vi "Variant to ITX Wave.vi"(8 "error in (no error)":errorcluster, 10 "Data":variant, 11 "Wavename":string) -> (0 "error out":errorcluster, 3 "ITX Wave":string)   [LabVIEW 2019, in "LV-Data.ITX.lvclass"]
uses:
  LV-Data.ITX.lvclass
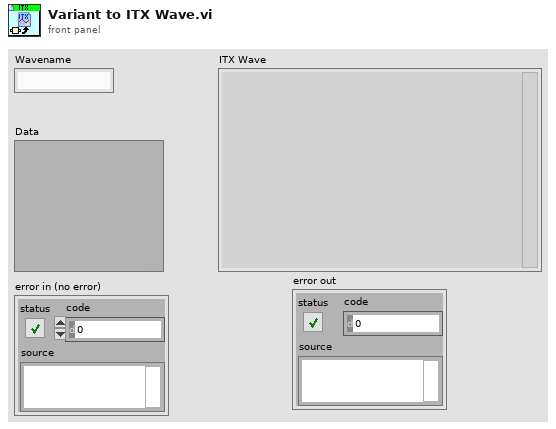
[diagram p1: front panel]
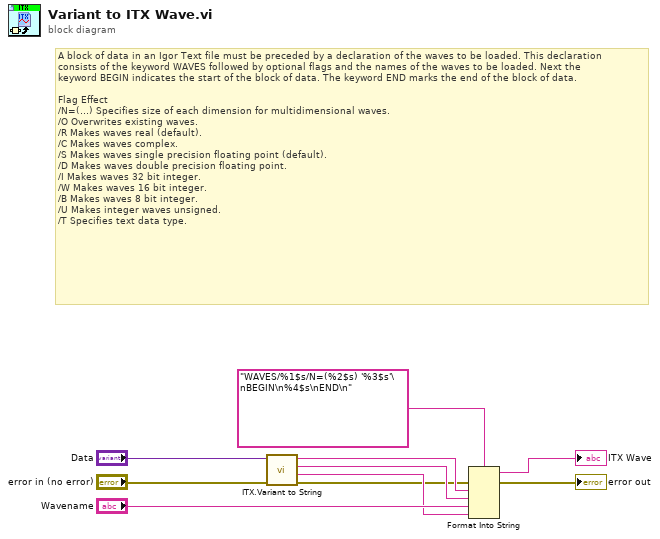
[diagram p0: block diagram]
diagram:
  # "A block of data in an Igor Text file must be preceded by a declaration of the waves to be loaded. This declaration\nconsists of the keyword WAVES followed by optional flags and the names of the waves to be loaded. Next the\nkeyword BEGIN indicates the start of the block of data. The keyword END marks the end of the block of data.\n\nFlag Effect\n/N=(…) Specifies size of each dimension for multidimensional waves.\n/O Overwrites existing waves.\n/R Makes waves real (default).\n/C Makes waves complex.\n/S Makes waves single precision floating point (default).\n/D Makes waves double precision floating point.\n/I Makes waves 32 bit integer.\n/W Makes waves 16 bit integer.\n/B Makes waves 8 bit integer.\n/U Makes integer waves unsigned.\n/T Specifies text data type."
  n1 = call "ITX.Variant to String.vi"("error in (no error)"="error in (no error)", "Data (Variant)"="Data") -> ("error out"=w1:errorcluster, "Data"=w2:string, "Size"=w3:string, "Type"=w4:string)  [unwired: 6 in]
  n2 = Format Into String(format string="WAVES/%1$s/N=(%2$s) '%3$s'\nBEGIN\n%4$s\nEND\n", error in=w1, w4, w3, "Wavename", w2) -> (resulting string=→"ITX Wave":string, error out=→"error out":errorcluster)  [unwired: 1 in]
